vi "runscenario Query with Result.vi"(6 "User":T5, 7 "Connection Refnum":T2, 8 "error in (no error)":errorcluster, 9 "Result FieldIds CSV (\"\")":string, 10 "Logic String (\"\": AND all conditions)":string, 11 "Conditions (none)":T3[](array[typedef])) -> (0 "error out":errorcluster, 2 "jsResults":string, 3 "runs":T1[](array[typedef]))   [LabVIEW 2011]
uses:
  server/database/Users/User Record.ctl
  server/database/Scenarios/Conditions/Condition Record.ctl
  server/database/Scenarios/Conditions/Condition Operators.ctl
  Summitek EXT/ODBC/SQL Controls/Connection Refnum.ctl
  _cgi-lib/TDM_INDEX Record.ctl
  server/DIAdem/lib/DIAdem Query Queue.ctl
  server/DataFinder/Datafinder Query.ctl
  server/DataFinder/eSearch Types.ctl
  server/DataFinder/DataFinder Comparisons.ctl
  server/database/Fields/Field Record.ctl
  server/database/Fields/Field DataTypes.ctl
  server/database/Fields/Field NextItem.ctl
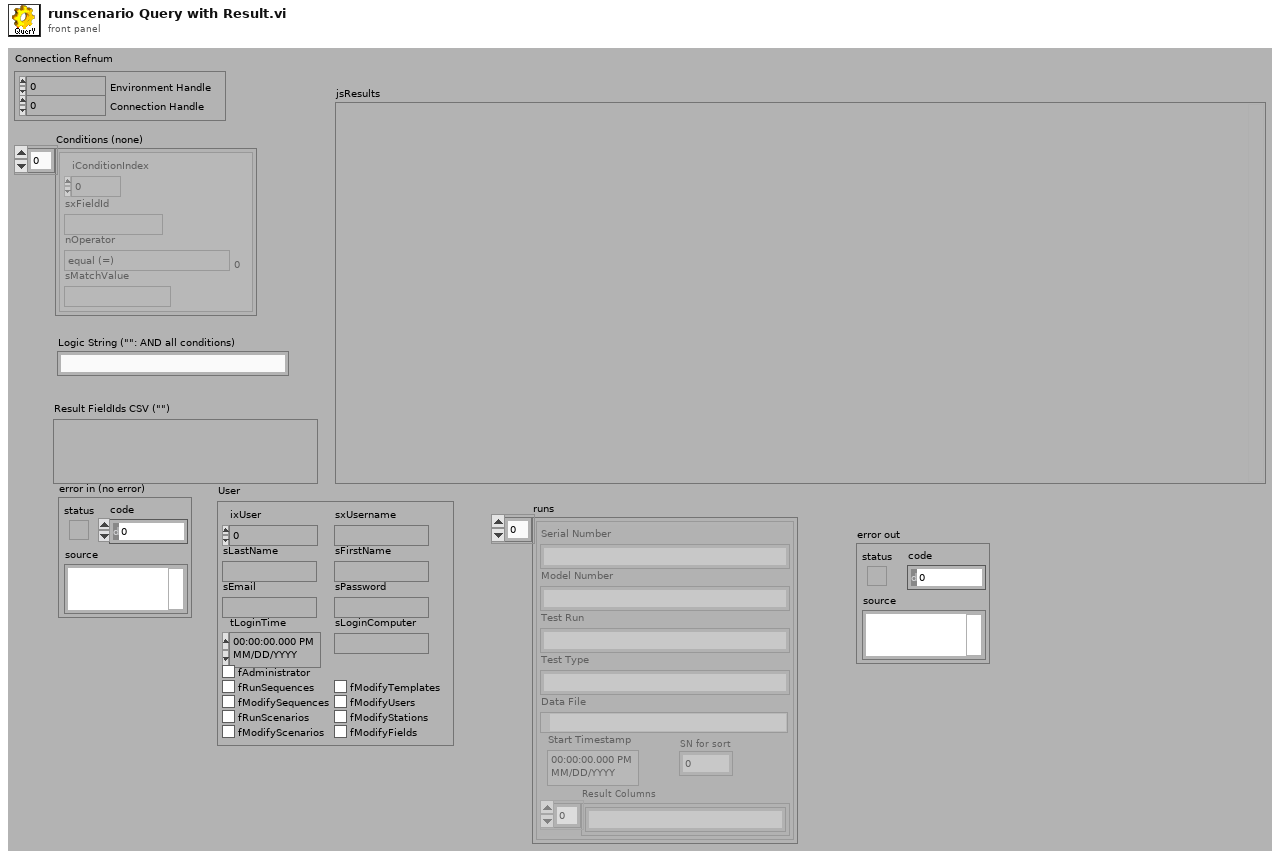
[diagram p1: front panel]
types:
  T1 = typedef "TDM_INDEX Record.ctl" = cluster{"Model Number":string, "SN for sort":i32, "Test Type":string, "Test Run":string, "Serial Number":string, "Start Timestamp":timestamp, "Data File":path, "Result Columns":string[]}
  T2 = typedef "Connection Refnum.ctl" = cluster{"Environment Handle":i32, "Connection Handle":i32}
  T3 = typedef "Condition Record.ctl" = cluster{"iConditionIndex":i32, "sxFieldId":string, "nOperator":T4, "sMatchValue":string}
  T4 = typedef "Condition Operators.ctl" = enum16{"equal (=)", "not equal (\\u2260)", "less than (<)", "less than or equal (\\u2264)", "greater than (>)", "greater than or equal (\\u2265)", "contains", "does not contain"}
  T5 = typedef "User Record.ctl" = cluster{"ixUser":i32, "sxUsername":string, "sLastName":string, "sFirstName":string, "sEmail":string, "sPassword":string, "tLoginTime":timestamp, "sLoginComputer":string, "fAdministrator":bool, "fRunSequences":bool, "fModifySequences":bool, "fRunScenarios":bool, "fModifyScenarios":bool, "fModifyTemplates":bool, "fModifyUsers":bool, "fModifyStations":bool, "fModifyFields":bool}
  T6 = typedef "DIAdem Query Queue.ctl" = cluster{"UserName":string, "Search Parameters":T7[], "eSearch Type":T8, "Query Name (vbs)":string, "Response queue name":string, "Logic String":string}
  T7 = typedef "Datafinder Query.ctl" = cluster{"eSearch Types":T8, "Property Name":string, "DataFinder Comparisons":T9, "Property Value":string}
  T8 = typedef "eSearch Types.ctl" = enum16{"eSearchFile", "eSearchChannelGroup", "eSearchChannel"}
  T9 = typedef "DataFinder Comparisons.ctl" = enum16{"=", "<>", "<", "<=", ">", ">="}
  T10 = typedef "Keyed Array.ctl" = cluster{"keys":string[], "values":string[]}
  T11 = typedef "Field Record.ctl" = cluster{"ixField":i32, "iSequenceOrder":i32, "sxFieldId":string, "sxSequenceId":string, "sDisplayName":string, "sValue":string, "sUnits":string, "nDataType":T12, "nNextItem":T13, "fSystem":bool, "fSystemValue":bool, "fRequired":bool, "fSetAtTest":bool, "fTestField":bool, "fDeleted":bool, "fIndexed":bool, "fFreeList":bool}
  T12 = typedef "Field DataTypes.ctl" = enum32{"text", "numeric", "list", "timestamp", "boolean"}
  T13 = typedef "Field NextItem.ctl" = enum32{"Reset", "Retain", "Auto-Increment"}
  T14 = cluster{"Items[0]":string, "Items[1]":string, "Items[2]":string, "Items[3]":string}
  T15 = typedef "TDMS File.ctl" = cluster{"File Path":path, "Run Data":T16[], "Serial Number":string, "Model Number":string, "Test Type":string}
  T16 = typedef "TDMS Run.ctl" = cluster{"Channel Data":T17[], "Custom Fields":T11[], "Run ID":string}
  T17 = typedef "TDMS Channel (Sxx).ctl" = cluster{"Channel Name":string, "Waveform":dbl[], "Unit":string, "List value":string}
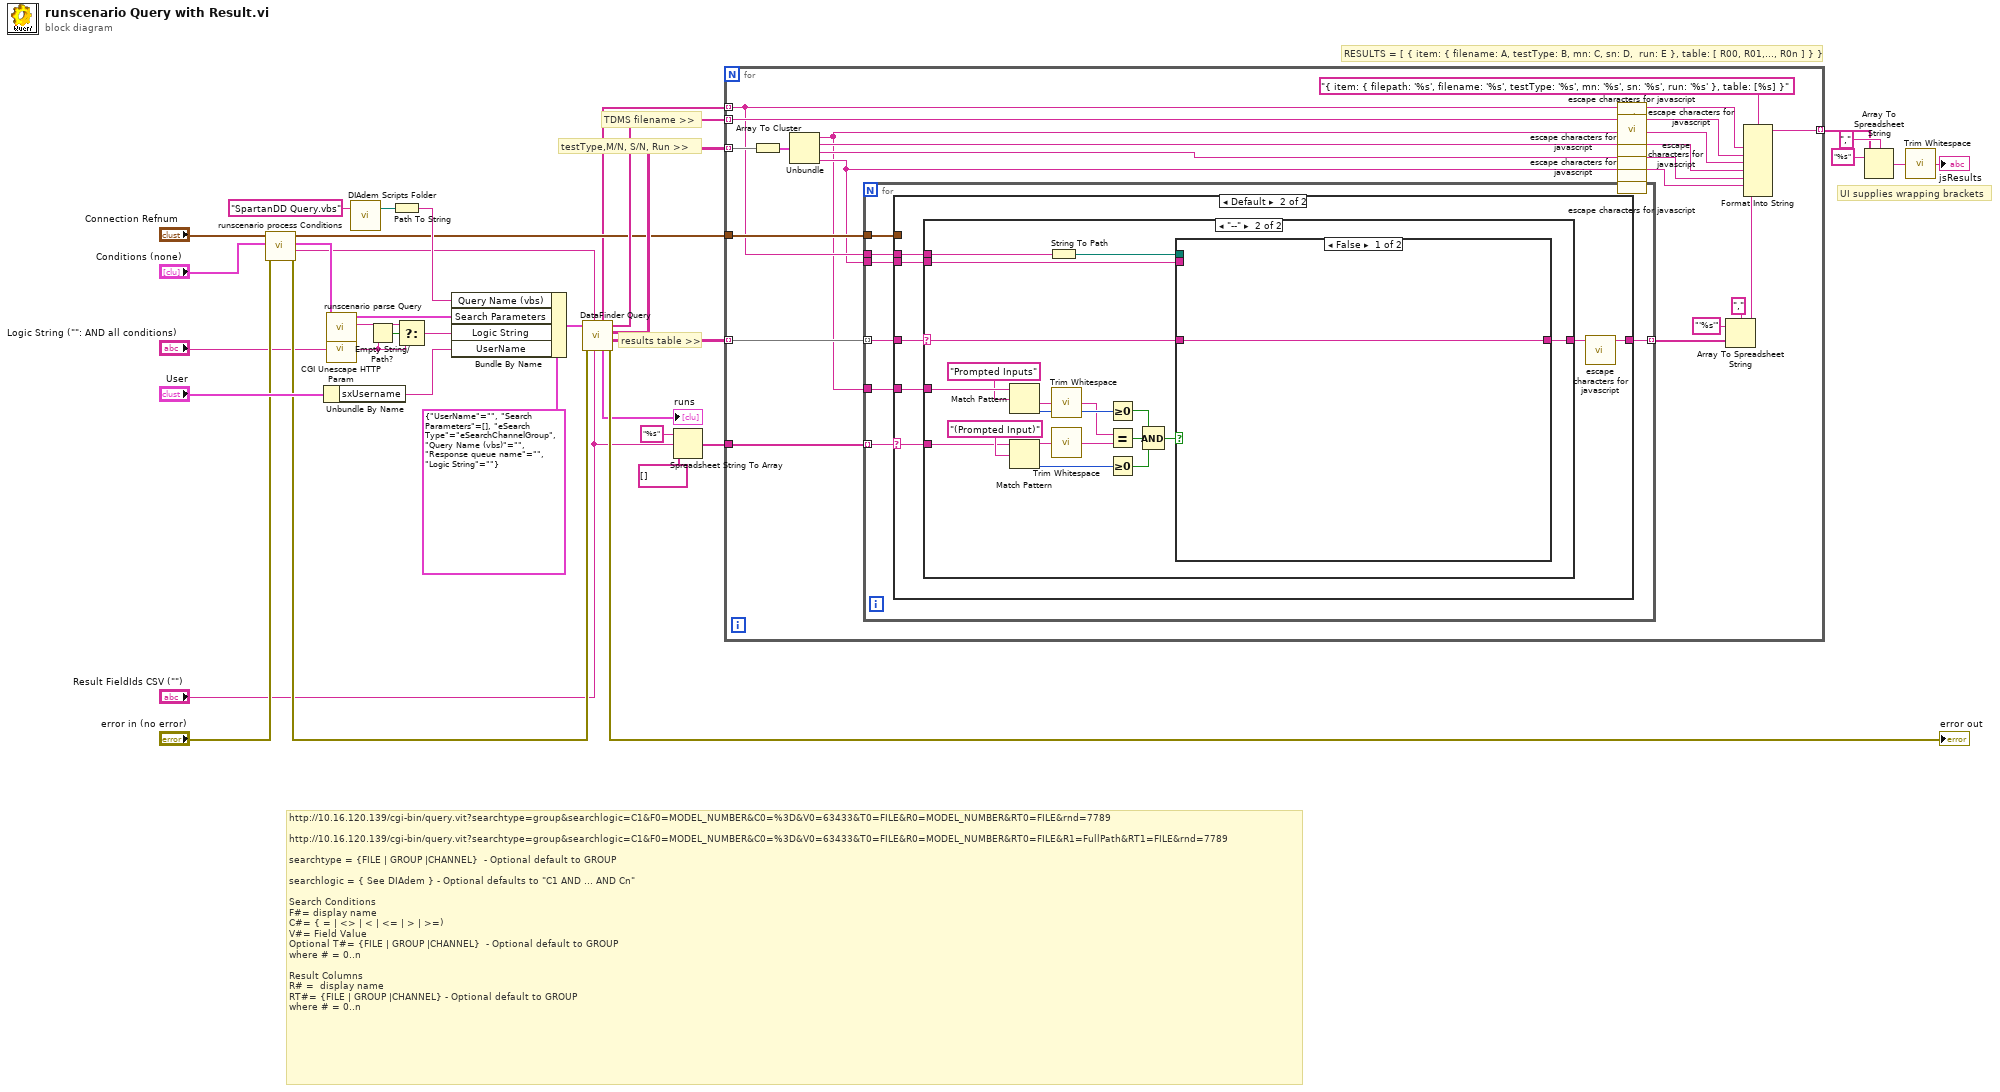
[diagram p0: block diagram]
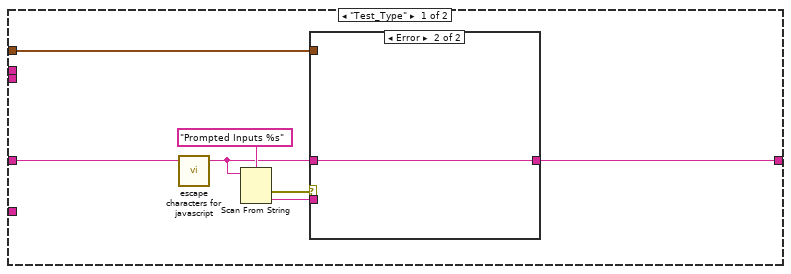
[diagram p2: hidden frame]
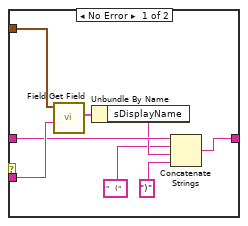
[diagram p3: hidden frame]
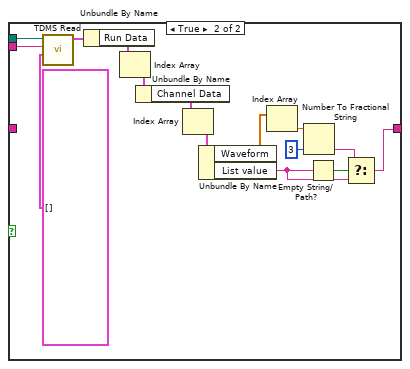
[diagram p5: hidden frame]
diagram:
  # "UI supplies wrapping brackets"
  # "TDMS filename >>"
  # "RESULTS = [ { item: { filename: A, testType: B, mn: C, sn: D,  run: E }, table: [ R00, R01,..., R0n ] } }"
  # "results table >>"
  # "testType,M/N, S/N, Run >>"
  # "http://10.16.120.139/cgi-bin/query.vit?searchtype=group&searchlogic=C1&F0=MODEL_NUMBER&C0=%3D&V0=63433&T0=FILE&R0=MODEL_NUMBER&RT0=FILE&rnd=7789\n\nhttp://10.16.120.139/cgi-bin/query.vit?searchtype=group&searchlogic=C1&F0=MODEL_NUMBER&C0=%3D&V0=63433&T0=FILE&R0=MODEL_NUMBER&RT0=FILE&R1=FullPath&RT1=FILE&rnd=7789\n\nsearchtype = {FILE | GROUP |CHANNEL}  - Optional default to GROUP \n\nsearchlogic = { See DIAdem } - Optional defaults to \"C1 AND ... AND Cn\"\n\nSearch Conditions\nF#= display name\nC#= { = | <> | < | <= | > | >=)\nV#= Field Value\nOptional T#= {FILE | GROUP |CHANNEL}  - Optional default to GROUP \nwhere # = 0..n\n\nResult Columns\nR# =  display name\nRT#= {FILE | GROUP |CHANNEL} - Optional default to GROUP \nwhere # = 0..n"
  n1 = call "runscenario process Conditions.vi"("error in (no error)"="error in (no error)", "Conditions (none)"="Conditions (none)", "Connection Refnum"="Connection Refnum") -> ("error out"=w19:errorcluster, "Test Run Filter"=w21:string, "Conditions"=w26:T10, "dup Connection Refnum"=w2:T2)  [unwired: 5 out]
  n2 = Unbundle By Name("User") -> ("sxUsername"=w29:string)
  n3 = call "runscenario parse Query.vi"("Query as Key/Value (empty)"=w26) -> ("ANDed Condition Logic"=w24:string, "Search Parameters"=w28:T7[])  [unwired: 4 in, 5 out]
  n4 = call "CGI Unescape HTTP Param.vi"("url-encoded string"="Logic String (\"\": AND all conditions)") -> ("string"=w16:string)
  n5 = call "DIAdem Scripts Folder.vi"("Relative Path (\"\" - Folder)"="SpartanDD Query.vbs" ("Property Name")) -> ("Scripts Folder"=w32:path)  [unwired: 2 out]
  n6 = Empty String/Path?(string/path=w16) -> (empty?=w25:bool)
  n7 = Path To String(path=w32) -> (string=w31:string)
  n8 = Select(t=w24, s=w25, f=w16) -> (s? t:f=w23:string)
  n9 = Bundle By Name(cluster=T6 {"UserName"="", "Search Parameters"=[], "eSearch Type"=enum."eSearchChannelGroup", "Query Name (vbs)"="", "Response queue name"="", "Logic String"=""} ("Query Request"), "Query Name (vbs)"=w31, "Search Parameters"=w28, "Logic String"=w23, "UserName"=w29) -> (w34:T6)
  n10 = call "DataFinder Query.vi"("result columns (comma list)"="Result FieldIds CSV (\"\")", "Run search type (\"\")"=w21, "error in (no error)"=w19, "Query Parameters"=w34) -> ("error out"=→"error out":errorcluster, "Results"=w11:string[][], "Items"=w10:string[][], "Item Filenames"=w9:string[], "runs"=→"runs":T1[], "Item Filepaths"=w1:string[])  [unwired: 2 in]
  n11 = Spreadsheet String To Array(format string="%s", spreadsheet string="Result FieldIds CSV (\"\")", array type (2D Dbl)=string[] []) -> (array=w3:string[])  [unwired: 1 out]
  n12 = for {
    tunnel: w11 -> [w45] mode=indexing
    tunnel: w9 -> [w57] mode=indexing
    tunnel: w10 -> [w56] mode=indexing
    tunnel: [w44] -> w12 mode=indexing
    tunnel: w3 -> [w41]
    tunnel: w2 -> [w42]
    tunnel: w1 -> [w38] mode=indexing
    n13 = Array To Cluster(array=w56) -> (cluster=w55:T14)
    n14 = Unbundle(w55) -> ("Items[0]"=w36:string, "Items[1]"=w54:string, "Items[2]"=w53:string, "Items[3]"=w37:string)
    n15 = for {
      tunnel: w45 -> [w65] mode=indexing
      tunnel: [w64] -> w46 mode=indexing
      tunnel: w42 -> [w63]
      tunnel: w41 -> [w62] mode=indexing
      tunnel: w38 -> [w61]
      tunnel: w37 -> [w60]
      tunnel: w36 -> [w59]
      n16 = case shown="Default" w62 {
        selector: w62 -> [_ w83]
        tunnel: w65 -> [w72 w87]
        tunnel: [w69 w88] -> w64
        tunnel: w63 -> [w66 _]
        tunnel: w61 -> [_ w85]
        tunnel: w60 -> [_ w84]
        tunnel: w59 -> [_ w82]
        frame "Test_Type" {
          n17 = call "escape characters for javascript.vi"("String (\"\")"=w72) -> ("escaped String"=w68:string)  [unwired: 4 out]
          n18 = Scan From String(format string="Prompted Inputs %s", input string=w68) -> (error out=w70:errorcluster, output 1=w67:string)  [unwired: 3 in, 2 out]
          n19 = case shown="Error" w70 {
            tunnel: [w77 w81] -> w69
            tunnel: w68 -> [w76 w81]
            tunnel: w67 -> [w80 _]
            tunnel: w66 -> [w79 _]
            frame No Error {
              n20 = call "Field Get Field.vi"("sFieldId or sDisplayName (\"\")"=w80, "Connection Refnum"=w79) -> ("Field"=w78:T11)  [unwired: 6 in, 3 out]
              n21 = Unbundle By Name(w78) -> ("sDisplayName"=w75:string)
              n22 = Concatenate Strings(w76, "   (" ("string"), w75, ")" ("string")) -> (w77:string)
            }
            frame Error {
            }
          }
        }
        frame Default {
          n23 = case shown="\"--\"" w87 {
            selector: w87 -> [w89 w103]
            tunnel: [w89 w105] -> w86
            tunnel: w85 -> [_ w108]
            tunnel: w84 -> [_ w107]
            tunnel: w83 -> [_ w102]
            tunnel: w82 -> [_ w99]
            frame Default {
            }
            frame "--" {
              n24 = Match Pattern(string=w99, regular expression="Prompted Inputs") -> (after substring=w96:string, offset past match=w100:i32)  [unwired: 1 in, 2 out]
              n25 = Match Pattern(string=w102, regular expression="(Prompted Input)") -> (before substring=w97:string, offset past match=w101:i32)  [unwired: 1 in, 2 out]
              n26 = String To Path(string=w108) -> (path=w106:path)
              n27 = call <vilib>:"Trim Whitespace.vi"("string"=w96) -> ("trimmed string"=w95:string)  [unwired: 1 in]
              n28 = call <vilib>:"Trim Whitespace.vi"("string"=w97) -> ("trimmed string"=w94:string)  [unwired: 1 in]
              n29 = Greater Or Equal To 0?(x=w100) -> (x >= 0?=w91:bool)
              n30 = Equal?(x=w95, y=w94) -> (x = y?=w90:bool)
              n31 = Greater Or Equal To 0?(x=w101) -> (x >= 0?=w92:bool)
              n32 = Compound Arithmetic op=AND(w91, w90, w92) -> (w93:bool)
              n33 = case shown="False" w93 {
                tunnel: w107 -> [_ w124]
                tunnel: w106 -> [_ w123]
                tunnel: [w109 w112] -> w105
                tunnel: w103 -> [w109 _]
                frame False {
                }
                frame True {
                  n34 = call "TDMS Read.vi"("System or ALL Combined Fields"=T11[] [], "Run String"=w124, "TDM File Path"=w123) -> ("File Information"=w122:T15)  [unwired: 6 in, 2 out]
                  n35 = Unbundle By Name(w122) -> ("Run Data"=w121:T16[])
                  n36 = Index Array(array=w121) -> (element=w120:T16)  [unwired: 1 in]
                  n37 = Unbundle By Name(w120) -> ("Channel Data"=w119:T17[])
                  n38 = Index Array(array=w119) -> (element=w118:T17)  [unwired: 1 in]
                  n39 = Unbundle By Name(w118) -> ("Waveform"=w115:dbl[], "List value"=w116:string)
                  n40 = Index Array(array=w115) -> (element=w113:dbl)  [unwired: 1 in]
                  n41 = Number To Fractional String(number=w113, precision (6)=i16 3) -> (F-format string=w114:string)  [unwired: 2 in]
                  n42 = Empty String/Path?(string/path=w116) -> (empty?=w117:bool)
                  n43 = Select(t=w114, s=w117, f=w116) -> (s? t:f=w112:string)
                }
              }
            }
          }
          n44 = call "escape characters for javascript.vi"("String (\"\")"=w86) -> ("escaped String"=w88:string)  [unwired: 4 out]
        }
      }
    }
    n45 = call "escape characters for javascript.vi"("String (\"\")"=w38) -> ("escaped String"=w39:string)  [unwired: 4 out]
    n46 = call "escape characters for javascript.vi"("String (\"\")"=w57) -> ("escaped String"=w40:string)  [unwired: 4 out]
    n47 = call "escape characters for javascript.vi"("String (\"\")"=w36) -> ("escaped String"=w52:string)  [unwired: 4 out]
    n48 = call "escape characters for javascript.vi"("String (\"\")"=w54) -> ("escaped String"=w51:string)  [unwired: 4 out]
    n49 = call "escape characters for javascript.vi"("String (\"\")"=w53) -> ("escaped String"=w50:string)  [unwired: 4 out]
    n50 = call "escape characters for javascript.vi"("String (\"\")"=w37) -> ("escaped String"=w49:string)  [unwired: 4 out]
    n51 = Array To Spreadsheet String(delimiter (Tab)=",", array=w46, 3:"'%s'" ("format string")) -> (spreadsheet string=w43:string)
    n52 = Format Into String(format string="{ item: { filepath: '%s', filename: '%s', testType: '%s', mn: '%s', sn: '%s', run: '%s' }, table: [%s] }", w39, w40, w52, w51, w50, w49, w43) -> (resulting string=w44:string)  [unwired: 2 in, 1 out]
  }
  n53 = Array To Spreadsheet String(delimiter (Tab)=",", array=w12, 3:"%s" ("format string")) -> (spreadsheet string=w15:string)
  n54 = call <vilib>:"Trim Whitespace.vi"("string"=w15) -> ("trimmed string"=→"jsResults":string)  [unwired: 1 in]
